vi "频率计（实采）.vi"() -> ()   [LabVIEW 2017]
uses:
  <vilib>/Analysis/4window.llb/windowTd.ctl
  <vilib>/DAQmx/read.llb/DAQmx Read (Analog Wfm 1Chan NSamp).vi
  <vilib>/DAQmx/create/channels.llb/DAQmx Create Channel (AI-Voltage-Basic).vi
  <vilib>/DAQmx/configure/timing.llb/DAQmx Timing (Sample Clock).vi
  <vilib>/DAQmx/miscellaneous.llb/DAQmx Fill In Error Info.vi
  <vilib>/measure/mascope.llb/Pulse Measurements 1 chan.vi
  <vilib>/measure/matone.llb/Extract Single Tone Information 1 Chan.vi
  <vilib>/measure/NI_MAPro.lvlib
  <vilib>/Analysis/NI_AALPro.lvlib
panel:
  in  "samples per channel":i32=1000 caption="每通道采样"
  in  "rate":dbl=1000.0 caption="采样率" format="%0.2f"
  out "波形图 2":waveform(dbl)(graph)
  out "FFTHanning窗校正":dbl
  out "FFT矩形窗校正":dbl
  out "三点法":dbl
  out "峰值多周期":dbl
  out "直流分量":dbl
  out "脉冲测量法":dbl
  out "过零插值":dbl
  out "过零多周期":dbl
  out "提取单频信息":dbl caption="检测到的频率" format="%.6p"
  out "FFT":dbl
  out "过零比较法":dbl
  out "波形图":waveform(dbl)(graph)
  # "频率计"
  # "时域算法"
  # "频域算法"
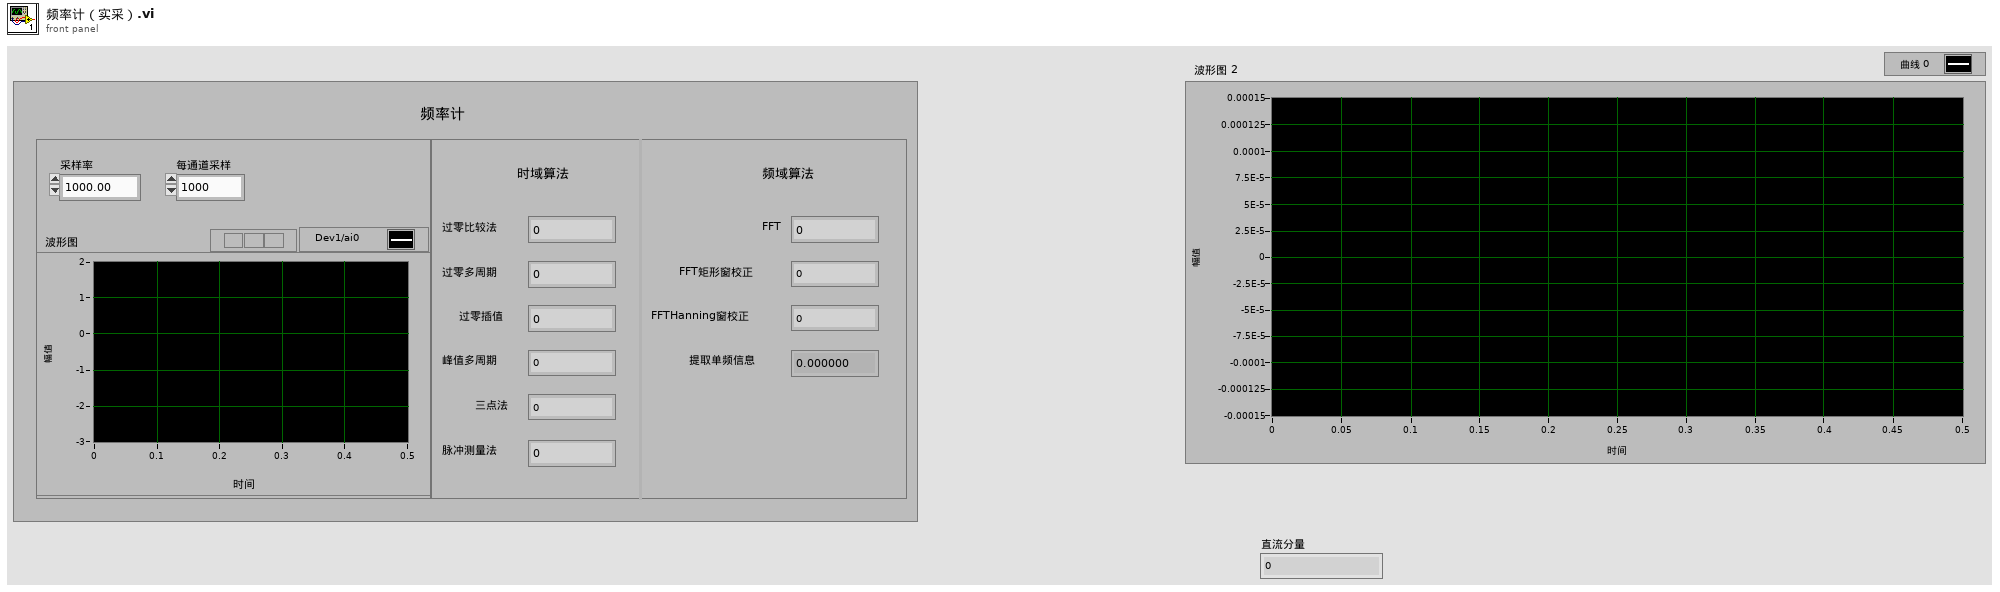
[diagram p1: front panel]
types:
  T1 = typedef "NI_AALPro.lvlib/windowTd.ctl" = u32
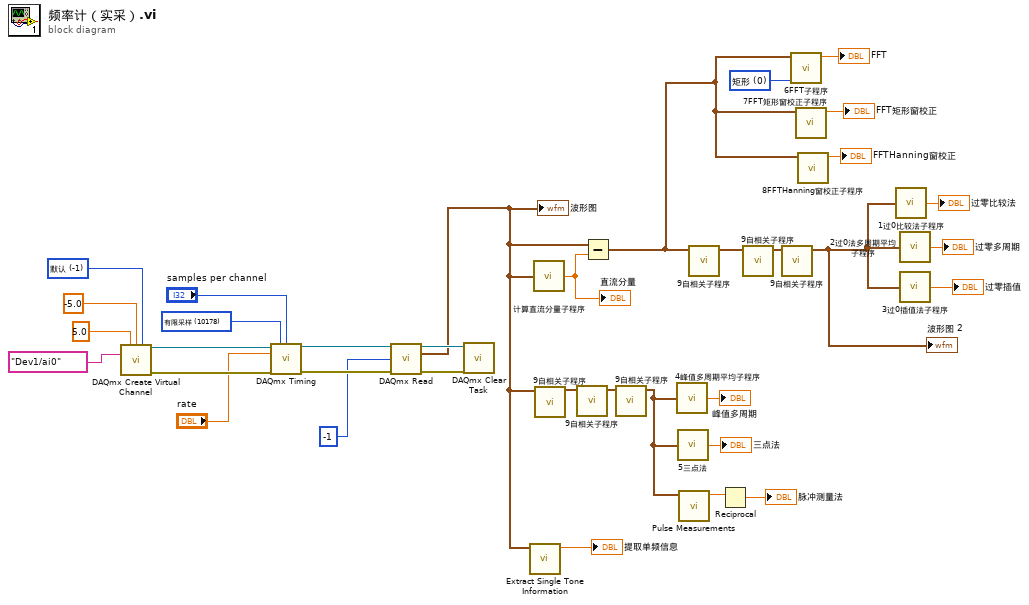
[diagram p0: block diagram]
diagram:
  w4 = 10178 items=["有限采样"=10178, "连续采样"=10123, "硬件定时单点"=12522] ("sample mode")
  w6 = -1 items=["默认"=-1, "RSE"=10083, "NRSE"=10078, "差分"=10106, "伪差分"=12529] ("input terminal configuration")
  w23 = T1 0 items=["矩形"=0, "Hanning"=1, "Hamming"=2, "Blackman-Harris"=3, "Exact Blackman"=4, "Blackman"=5, "Flat Top"=6, "4阶Blackman-Harris "=7, "7阶Blackman-Harris"=8, "Low Sidelobe"=9, "Blackman Nuttall"=11, "三角"=30, "Bartlett-Hanning"=31, "Bohman"=32, "Parzen"=33, "Welch"=34, "Kaiser"=60, "Dolph-Chebyshev"=61, "高斯"=62] ("window")
  n1 = call-poly <vilib>:"DAQmx Create Virtual Channel.vi"("maximum value"=5.0, "minimum value"=-5.0, "input terminal configuration"=w6, "physical channels"=tag "Dev1/ai0") -> ("task out"=w15:refnum<k21>, "error out"=w12:errorcluster)  [unwired: 10 in]
  n2 = call-poly <vilib>:"DAQmx Timing.vi"("task/channels in"=w15, "sample mode"=w4, "samples per channel"="samples per channel", "rate"="rate", "error in"=w12) -> ("task out"=w14:refnum<k21>, "error out"=w11:errorcluster)  [unwired: 9 in]
  n3 = call-poly <vilib>:"DAQmx Read.vi"("task/channels in"=w14, "number of samples per channel"=-1, "error in"=w11) -> ("task out"=w13:refnum<k21>, "data"=w1:waveform(dbl), "error out"=w10:errorcluster)  [unwired: 10 in]
  "波形图" <- w1
  n4 = call <vilib>:"DAQmx Clear Task.vi"("task in"=w13, "error in"=w10) -> ()  [unwired: 13 in, 1 out]
  n5 = call-poly <vilib>:"Extract Single Tone Information.vi"("time signal in"=w1) -> ("detected frequency"=→"提取单频信息":dbl)  [unwired: 5 in, 5 out]
  n6 = call "计算直流分量子程序.vi"("波形"=w1) -> ("直流分量"=w28:dbl)
  "直流分量" <- w28
  n7 = call "9自相关子程序.vi"("time signal"=w1) -> ("波形图"=w17:waveform(dbl))  [unwired: 6 in]
  n8 = call "9自相关子程序.vi"("time signal"=w17) -> ("波形图"=w18:waveform(dbl))  [unwired: 6 in]
  n9 = Subtract(x=w1, y=w28) -> (x-y=w22:waveform(dbl))
  n10 = call "9自相关子程序.vi"("time signal"=w18) -> ("波形图"=w16:waveform(dbl))  [unwired: 6 in]
  n11 = call "4峰值多周期平均子程序.vi"("波形"=w16) -> ("f"=→"峰值多周期":dbl)
  n12 = call "5三点法.vi"("波形"=w16) -> ("f"=→"三点法":dbl)
  n13 = call-poly <vilib>:"Pulse Measurements.vi"("signal in"=w16) -> ("period"=w30:dbl)  [unwired: 6 in, 4 out]
  n14 = call "9自相关子程序.vi"("time signal"=w22) -> ("波形图"=w21:waveform(dbl))  [unwired: 6 in]
  n15 = Reciprocal(x=w30) -> (1/x=→"脉冲测量法":dbl)
  n16 = call "9自相关子程序.vi"("time signal"=w21) -> ("波形图"=w20:waveform(dbl))  [unwired: 6 in]
  n17 = call "9自相关子程序.vi"("time signal"=w20) -> ("波形图"=w19:waveform(dbl))  [unwired: 6 in]
  "波形图 2" <- w19
  n18 = call "6FFT子程序.vi"("window"=w23, "time signal"=w22) -> ("频率"=→"FFT":dbl)  [unwired: 2 in, 3 out]
  n19 = call "7FFT矩形窗校正子程序.vi"("time signal"=w22) -> ("频率"=→"FFT矩形窗校正":dbl)  [unwired: 4 in, 2 out]
  n20 = call "8FFTHanning窗校正子程序.vi"("time signal"=w22) -> ("频率"=→"FFTHanning窗校正":dbl)  [unwired: 4 in, 2 out]
  n21 = call "1过0比较法子程序.vi"("波形"=w19) -> ("f"=→"过零比较法":dbl)
  n22 = call "2过0法多周期平均子程序.vi"("波形"=w19) -> ("f"=→"过零多周期":dbl)
  n23 = call "3过0插值法子程序.vi"("波形"=w19) -> ("f"=→"过零插值":dbl)
